vi "Process Data.vi"(0 "LD Reading in":refnum<class "LD Reading.lvclass">, 1 "reference":refnum<vi>, 4 "Input Cluster":T2) -> (22 "Realtime Output":T3, 23 "Output Cluster":T1)   [LabVIEW 2017, in "LD Reading.lvclass"]
uses:
  LD Reading.lvclass
  Realtime Output.ctl
  LD Reading.lvclass/LD Reading.ctl
panel:
  out "PMT Voltage (V)":cluster{dbl[], dbl[]}(graph)
  out "RMS Voltage (mV)":cluster{dbl[], dbl[]}(graph)
  out "Diode/PMT":cluster{dbl[], dbl[]}(graph)
  out "Photodiode Voltage  (V)":cluster{dbl[], dbl[]}(graph)
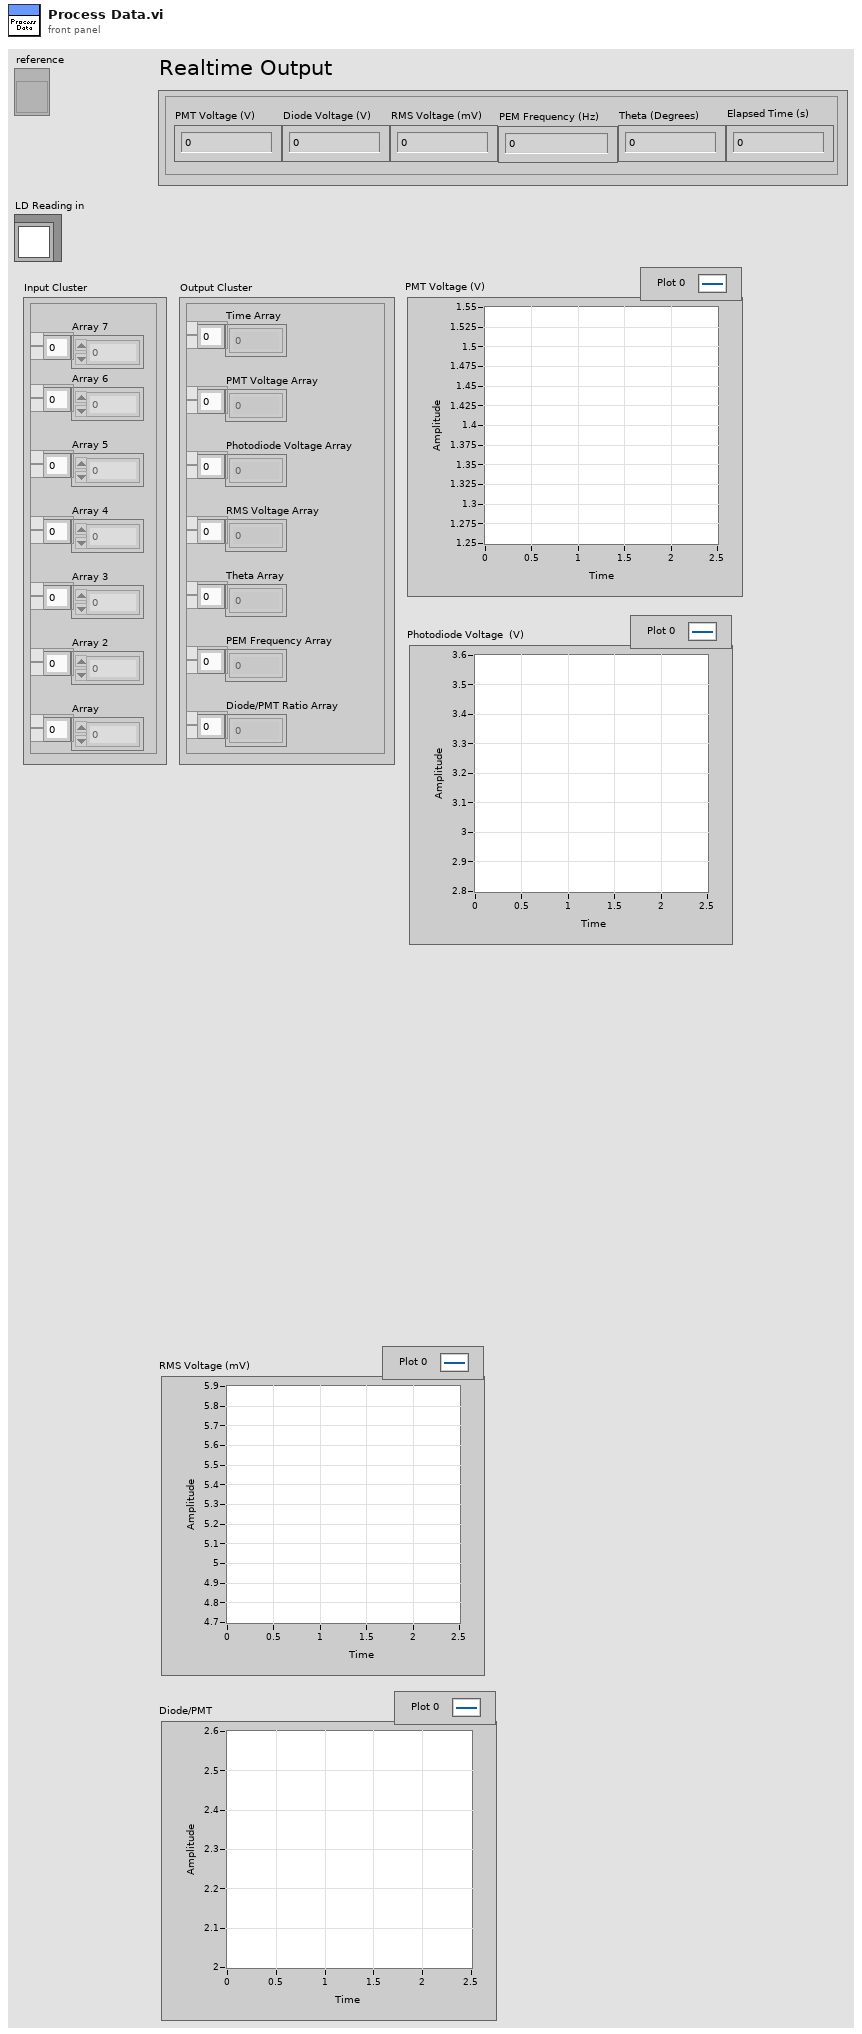
[diagram p1: front panel]
types:
  T1 = cluster{"RMS Voltage Array":dbl[], "Photodiode Voltage Array":dbl[], "PMT Voltage Array":dbl[], "Diode/PMT Ratio Array":dbl[], "Time Array":dbl[], "PEM Frequency Array":dbl[], "Theta Array":dbl[]}
  T2 = cluster{"Array 7":dbl[], "Array":dbl[], "Array 2":dbl[], "Array 3":dbl[], "Array 4":dbl[], "Array 5":dbl[], "Array 6":dbl[]}
  T3 = typedef "Realtime Output.ctl" = cluster{"Elapsed Time (s)":dbl, "PMT Voltage (V)":dbl, "Diode Voltage (V)":dbl, "RMS Voltage (mV)":dbl, "Theta (Degrees)":dbl, "PEM Frequency (Hz)":dbl}
  T4 = cluster{dbl[], dbl[], dbl[], dbl[], dbl[], dbl[], dbl[]}
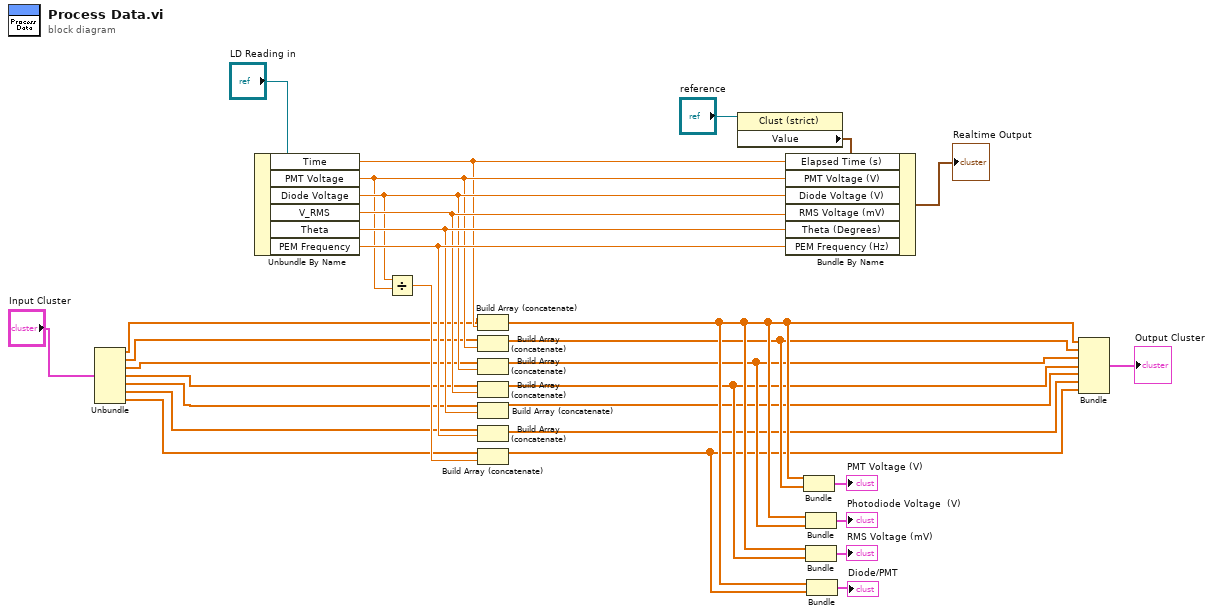
[diagram p0: block diagram]
diagram:
  n1 = Unbundle("Input Cluster") -> ("Array 7"=w15:dbl[], "Array"=w14:dbl[], "Array 2"=w13:dbl[], "Array 3"=w12:dbl[], "Array 4"=w11:dbl[], "Array 5"=w10:dbl[], "Array 6"=w9:dbl[])
  n2 = Unbundle By Name("LD Reading in") -> ("Time"=w25:dbl, "PMT Voltage"=w26:dbl, "Diode Voltage"=w27:dbl, "V_RMS"=w28:dbl, "Theta"=w29:dbl, "PEM Frequency"=w30:dbl)
  n3 = Divide(x=w27, y=w26) -> (x/y=w21:dbl)
  n4 = Build Array (concatenate)(w15, w25) -> (w8:dbl[])
  n5 = Build Array (concatenate)(w14, w26) -> (w7:dbl[])
  n6 = Build Array (concatenate)(w13, w27) -> (w6:dbl[])
  n7 = Build Array (concatenate)(w12, w28) -> (w5:dbl[])
  n8 = Build Array (concatenate)(w11, w29) -> (w4:dbl[])
  n9 = Build Array (concatenate)(w10, w30) -> (w3:dbl[])
  n10 = Build Array (concatenate)(w9, w21) -> (w2:dbl[])
  n11 = property class="Clust (strict)"(reference="reference") -> ("Value"=w31:T3)  [unwired: 1 in, 2 out]
  n12 = Bundle By Name(cluster=w31, "Elapsed Time (s)"=w25, "PMT Voltage (V)"=w26, "Diode Voltage (V)"=w27, "RMS Voltage (mV)"=w28, "Theta (Degrees)"=w29, "PEM Frequency (Hz)"=w30) -> (→"Realtime Output":T3)
  n13 = Bundle(w8, w7) -> (→"PMT Voltage (V)":cluster{dbl[], dbl[]})  [unwired: 1 in]
  n14 = Bundle(w8, w6) -> (→"Photodiode Voltage  (V)":cluster{dbl[], dbl[]})  [unwired: 1 in]
  n15 = Bundle(w8, w5) -> (→"RMS Voltage (mV)":cluster{dbl[], dbl[]})  [unwired: 1 in]
  n16 = Bundle(w8, w2) -> (→"Diode/PMT":cluster{dbl[], dbl[]})  [unwired: 1 in]
  n17 = Bundle(w8, w7, w6, w5, w4, w3, w2) -> (→"Output Cluster":T4)  [unwired: 1 in]
